vi "XLP80_CAN_FCCU_Errors.vi"(7 "Function":string, 8 "err in":errorcluster caption="error") -> (0 "err out":errorcluster caption="error", 2 "FCCU_Names":string[](array[string]), 3 "FCCU Errors":bool[](array[boolean]))   [LabVIEW 2021]
uses:
  XLP80_FGlob/1886_FGlob_TDefs_Enum_FGlobItems.ctl
  XLP80_Globals/XLP80_Globals_Status.vi
  XLP80_Globals/Globals_Settings_XLP80.vi
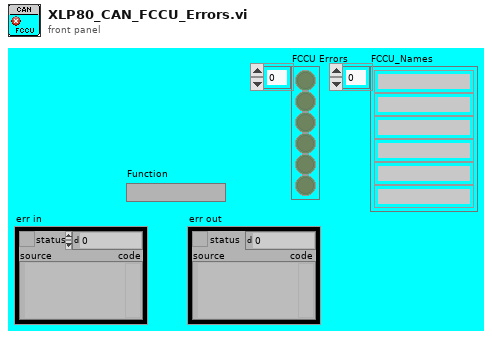
[diagram p1: front panel]
types:
  T1 = typedef "1886_FGlob_TDefs_Enum_FGlobItems.ctl" = enum16{"Put one", "Put all", "Recall one", "Recall all"}
  T2 = typedef "XLP80_Action_TDefEnumControl.ctl" = enum16{"Testmode_A", "Testmode_B"}
  T3 = cluster{"Signal Name":string[], "Description":string[], "Unit":string[], "Min":dbl[], "Max":dbl[], "HV & Software":bool[], "Basis Funktion":bool[], "Power Management":bool[], "OperationMode":bool[], "Shutdown":bool[], "Alarm":bool[], "LogEnable":bool[]}
  T4 = cluster{"Signal Name":string[], "Description":string[], "Unit":string[], "Min":dbl[], "Max":dbl[], "TestmodeA":bool[], "LogEnable":bool[]}
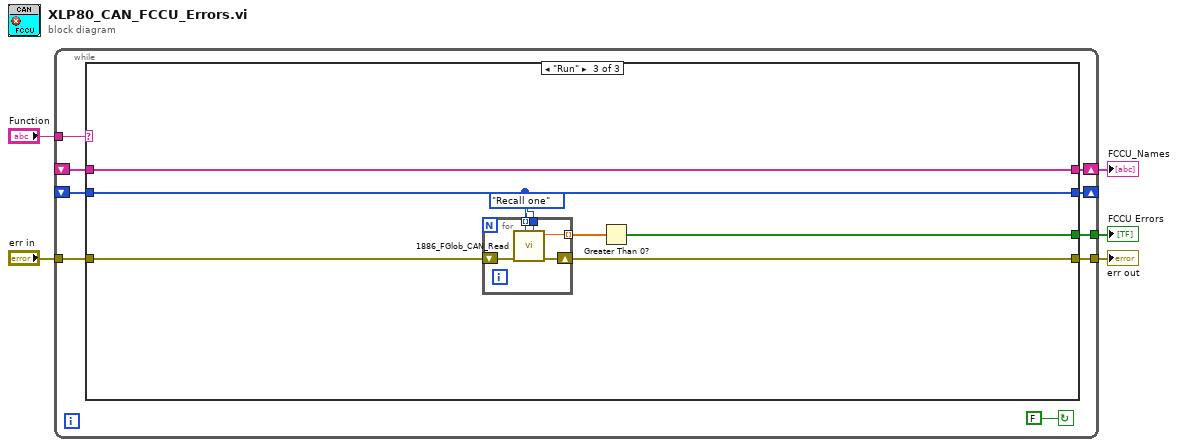
[diagram p0: block diagram]
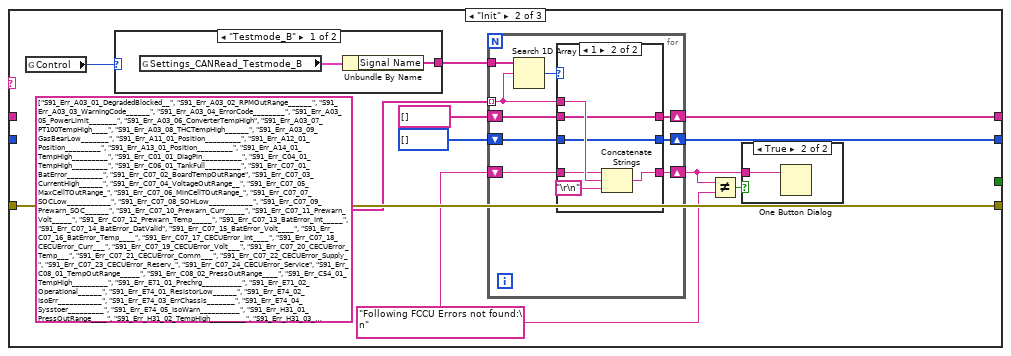
[diagram p3: hidden frame]
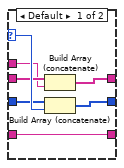
[diagram p4: hidden frame]
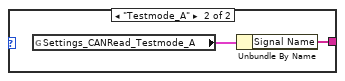
[diagram p6: hidden frame]
diagram:
  n1 = while {
    tunnel: "Function" -> [w13]
    tunnel: "err in" -> [w12]
    shift-right: [w9] -> _
    shift-left: _ -> [w11]
    tunnel: [w10] -> w3
    shift-right: [w8] -> w1
    shift-left: _ -> [w7]
    tunnel: [w6] -> w2
    stop <- FALSE continue-if-true
    n2 = case shown="\"Run\"" w13 {
      tunnel: w12 -> [w17 w27 w62]
      tunnel: w11 -> [w16 _ w59]
      tunnel: [w17 w27 w60] -> w10
      tunnel: [w16 w21 w59] -> w9
      tunnel: [w15 w18 w57] -> w8
      tunnel: w7 -> [w15 _ w57]
      tunnel: [_ _ w56] -> w6
      frame Default {
      }
      frame "Init" {
        w23 = "Following FCCU Errors not found:\n" ("string")
        n3 = global read "XLP80_Globals_Status.vi" "Control"() -> (w28:T2)
        n4 = case shown="\"Testmode_B\"" w28 {
          tunnel: [w52 w54] -> w26
          frame "Testmode_B" {
            n5 = global read "Globals_Settings_XLP80.vi" "Settings_CANRead_Testmode_B"() -> (w53:T3)
            n6 = Unbundle By Name(w53) -> ("Signal Name"=w52:string[])
          }
          frame "Testmode_A" {
            n7 = global read "Globals_Settings_XLP80.vi" "Settings_CANRead_Testmode_A"() -> (w55:T4)
            n8 = Unbundle By Name(w55) -> ("Signal Name"=w54:string[])
          }
        }
        n9 = for {
          tunnel: w26 -> [w37]
          tunnel: string[] ["S91_Err_A03_01_DegradedBlocked__", "S91_Err_A03_02_RPMOutRange______", "S91_Err_A03_03_WarningCode______", "S91_Err_A03_04_ErrorCode________", "S91_Err_A03_05_PowerLimit_______", "S91_Err_A03_06_ConverterTempHigh", "S91_Err_A03_07_PT100TempHigh____", "S91_Err_A03_08_THCTempHigh______", "S91_Err_A03_09_GasBearLow_______", "S91_Err_A11_01_Position_________", "S91_Err_A12_01_Position_________", "S91_Err_A13_01_Position_________", "S91_Err_A14_01_TempHigh_________", "S91_Err_C01_01_DiagPin__________", "S91_Err_C04_01_TempHigh_________", "S91_Err_C06_01_TankFull_________", "S91_Err_C07_01_BatError_________", "S91_Err_C07_02_BoardTempOutRange", "S91_Err_C07_03_CurrentHigh______", "S91_Err_C07_04_VoltageOutRange__", "S91_Err_C07_05_MaxCellTOutRange_", "S91_Err_C07_06_MinCellTOutRange_", "S91_Err_C07_07_SOCLow___________", "S91_Err_C07_08_SOHLow___________", "S91_Err_C07_09_Prewarn_SOC______", "S91_Err_C07_10_Prewarn_Curr_____", "S91_Err_C07_11_Prewarn_Volt_____", "S91_Err_C07_12_Prewarn_Temp_____", "S91_Err_C07_13_BatError_Int_____", "S91_Err_C07_14_BatError_DatValid", "S91_Err_C07_15_BatError_Volt____", "S91_Err_C07_16_BatError_Temp____", "S91_Err_C07_17_CECUError_Int____", "S91_Err_C07_18_CECUError_Curr___", "S91_Err_C07_19_CECUError_Volt___", "S91_Err_C07_20_CECUError_Temp___", "S91_Err_C07_21_CECUError_Comm___", "S91_Err_C07_22_CECUError_Supply_", "S91_Err_C07_23_CECUError_Reserv_", "S91_Err_C07_24_CECUError_Service", "S91_Err_C08_01_TempOutRange_____", "S91_Err_C08_02_PressOutRange____", "S91_Err_C54_01_TempHigh_________", "S91_Err_E71_01_Prechrg__________", "S91_Err_E71_02_Operational______", "S91_Err_E74_01_ResistorLow______", "S91_Err_E74_02_IsoErr___________", "S91_Err_E74_03_ErrChassis_______", "S91_Err_E74_04_Sysstoer_________", "S91_Err_E74_05_IsoWarn__________", "S91_Err_H31_01_PressOutRange____", "S91_Err_H31_02_TempHigh_________", "S91_Err_H31_03_PressHigh________", "S91_Err_H36_01_Timeout__________", "S91_Err_H36_02_PressHigh________", "S91_Err_H40_01_Timeout__________", "S91_Err_H40_02_PressHigh________", "S91_Err_H42_01_SysStateErr______", "S91_Err_H42_02_MtrNTCFlr_DrCnd__", "S91_Err_H42_03_Mtr_Temp_Err_____", "S91_Err_H42_04_Mtr_Temp_DrCnd___", "S91_Err_H42_05_BrdgDrv_VCC_UVErr", "S91_Err_H42_06_ShortToGround_Err", "S91_Err_H42_07_ShortToBat_Err___", "S91_Err_H42_08_E2E_Err__________", "S91_Err_H42_09_SpdLimitRq_Err___", "S91_Err_H42_10_Blocked_Err______", "S91_Err_H42_11_Batt_Vltg_Err____", "S91_Err_H42_12_ECU_Temp_Err_____", "S91_Err_H42_13_ECU_Temp_DrCnd___", "S91_Err_H42_20_KNF_Error________", "S91_Err_H45_01_TankFull_________", "S91_Err_H51_01_LowCellVoltLow___", "S91_Err_H51_02_TotalVoltOutRange", "S91_Err_H51_03_StartVoltTimeout_", "S91_Err_H51_04_StopVoltTimeout__", "S91_Err_H53_01_StartTimeout_____", "S91_Err_H55_01_PressHigh________", "S91_Err_H62_01_ErrCode__________", "S91_Err_H62_02_ConcentratMax____", "S91_Err_H62_03_ConcentratHigh___", "S91_Err_H63_01_ErrCode__________", "S91_Err_H63_02_ConcentratMax____", "S91_Err_H63_03_ConcentratHigh___", "S91_Err_S91_01_LabviewErr_______"] ("array w/ subset deleted") -> [w31] mode=indexing
          shift-right: [w34] -> w21
          shift-left: i32[] [] -> [w35]
          shift-right: [w32] -> w20
          shift-left: w23 -> [w33]
          shift-right: [w29] -> w18
          shift-left: string[] [] -> [w30]
          n10 = Search 1D Array(1D array=w37, element=w31) -> (index of element=w36:i32)  [unwired: 1 in]
          n11 = case shown="1" w36 {
            selector: w36 -> [w44 _]
            tunnel: w35 -> [w43 w47]
            tunnel: [w42 w47] -> w34
            tunnel: w33 -> [w41 w48]
            tunnel: [w41 w46] -> w32
            tunnel: w31 -> [w39 w50]
            tunnel: w30 -> [w40 w45]
            tunnel: [w38 w45] -> w29
            frame Default {
              n12 = Build Array (concatenate)(w40, w39) -> (w38:string[])
              n13 = Build Array (concatenate)(w43, w44) -> (w42:i32[])
            }
            frame 1 {
              n14 = Concatenate Strings(w48, w50, "\r\n") -> (w46:string)
            }
          }
        }
        n15 = Not Equal?(x=w20, y=w23) -> (x != y?=w22:bool)
        n16 = case shown="True" w22 {
          tunnel: w20 -> [_ w51]
          frame False {
          }
          frame True {
            n17 = One Button Dialog(message=w51) -> ()  [unwired: 1 in, 1 out]
          }
        }
      }
      frame "Run" {
        n18 = for {
          tunnel: 1886_FGlob_TDefs_Enum_FGlobItems."Recall one" ("Function (Recall One)") -> [w66]
          shift-right: [w65] -> w60
          shift-left: w62 -> [w67]
          tunnel: w59 -> [w64] mode=indexing
          tunnel: [w63] -> w58 mode=indexing
          n19 = call "1886_FGlob_CAN_Read.vi"("Function (Recall One)"=w66, "CAN Read Items"=w64, "err in"=w67) -> ("err out"=w65:errorcluster, "AI Value OUT"=w63:dbl)  [unwired: 6 in, 1 out]
        }
        n20 = Greater Than 0?(x=w58) -> (x > 0?=w56:bool[])
      }
    }
  }
  "err out" <- w3
  "FCCU Errors" <- w2
  "FCCU_Names" <- w1
